vi "LJM_eAddresses2D.vi"(0 "Handle In":i32, 1 "NumFrames (Auto-Detect)":i32=-1, 5 "aAddresses":i32[](array[numeric]), 7 "aTypes":i32[](array[numeric]), 9 "aValuesIn":dbl[][](array[numeric]) format="%.2f", 11 "error in":errorcluster, 12 "aWrites":i32[](array[ring]) items=["Read", "Write"], 13 "aNumValues":i32[](array[numeric])) -> (4 "Handle Out":i32, 10 "aValuesOut":dbl[][](array[numeric]) format="%.2f", 14 "ErrorAddress":i32, 15 "error out":errorcluster)   [LabVIEW 2020]
uses:
  Library/Frameworks/LabJackM.framework
panel:
  # "1/20/2015:  Default value of NumFrames changed to -1 which\nequates to Auto-Detect.  If NumFrames = -1, then the NumFrames\ncontrol is ignored and the size of aNames/aAddresses is used to\ndetermine how many frames there are."
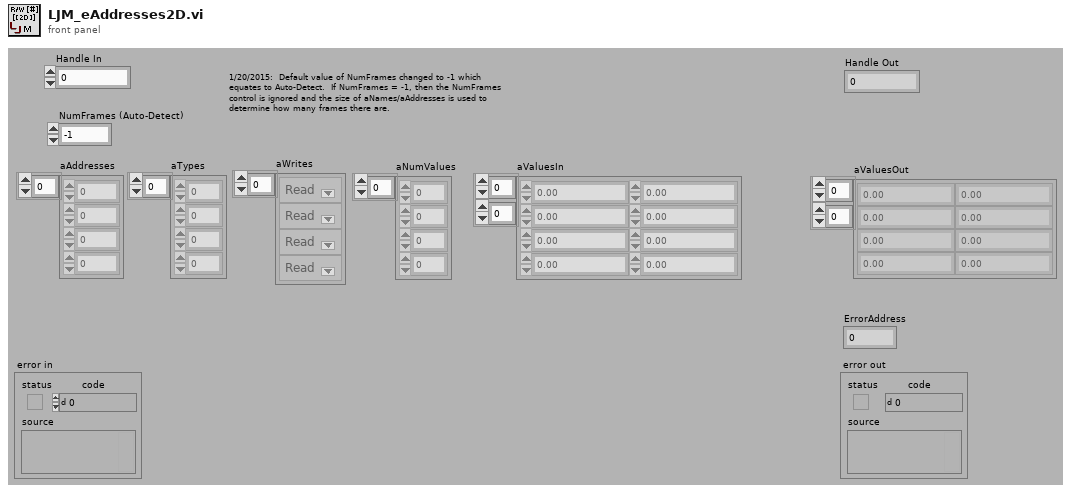
[diagram p1: front panel]
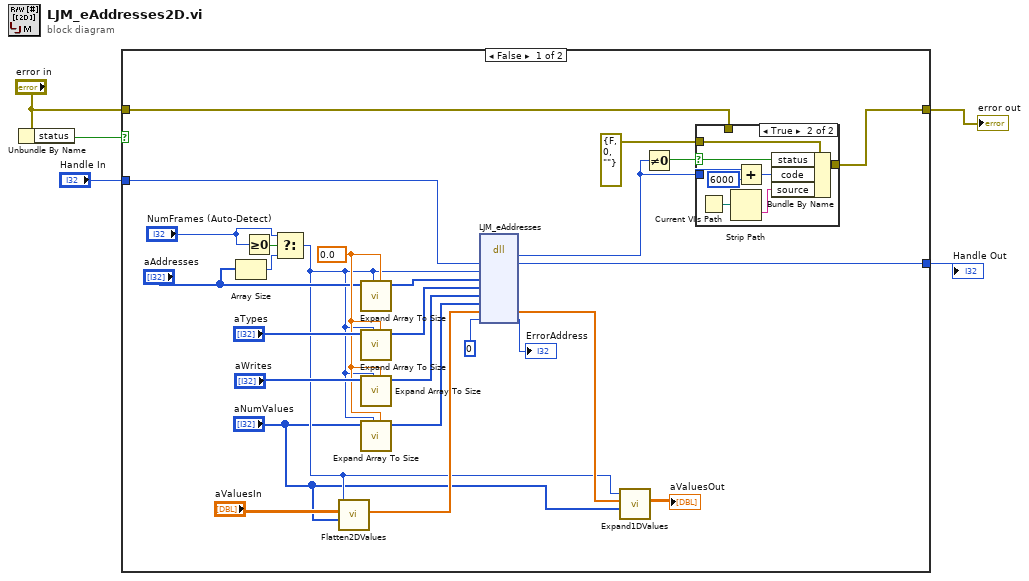
[diagram p0: block diagram]
diagram:
  n1 = Unbundle By Name("error in") -> ("status"=w5:bool)
  n2 = case shown="False" w5 {
    tunnel: "error in" -> [w28 w42]
    tunnel: [w27 w42] -> w3
    tunnel: [w13 w41] -> w2
    tunnel: "Handle In" -> [w12 w41]
    frame False {
      w18 = 0.0 ("Default Value")
      n3 = Array Size(array="aAddresses") -> (size(s)=w11:i32)
      n4 = Greater Or Equal To 0?(x="NumFrames (Auto-Detect)") -> (x >= 0?=w10:bool)
      n5 = Select(t="NumFrames (Auto-Detect)", s=w10, f=w11) -> (s? t:f=w7:i32)
      n6 = call "Flatten2DValues.vi"("NumValues"="aNumValues", "Values 2D"="aValuesIn", "NumFrames"=w7) -> ("Values 1D"=w16:dbl[])  [unwired: 8 in]
      n7 = call "Expand Array To Size.vi"("Default Value"=w18, "# Elements"=w7, "I32 Array In"="aAddresses") -> ("I32 Array Out"=w26:i32[])  [unwired: 4 in, 4 out]
      n8 = call "Expand Array To Size.vi"("Default Value"=w18, "# Elements"=w7, "I32 Array In"="aTypes") -> ("I32 Array Out"=w24:i32[])  [unwired: 4 in, 4 out]
      n9 = call "Expand Array To Size.vi"("Default Value"=w18, "# Elements"=w7, "I32 Array In"="aWrites") -> ("I32 Array Out"=w22:i32[])  [unwired: 4 in, 4 out]
      n10 = call "Expand Array To Size.vi"("Default Value"=w18, "# Elements"=w7, "I32 Array In"="aNumValues") -> ("I32 Array Out"=w21:i32[])  [unwired: 4 in, 4 out]
      n11 = dll-call lib="Library/Frameworks/LabJackM.framework" fn="LJM_eAddresses"("Handle"=w12, "NumFrames"=w7, "aAddresses"=w26, "aTypes"=w24, "aWrites"=w22, "aNumValues"=w21, "aValues"=w16, "ErrorFrame"=u32 0) -> ("return type"=w31:i32, "Handle"=w13:i32, "aValues"=w15:dbl[], "ErrorFrame"=→"ErrorAddress":i32)  [unwired: 8 in, 2 out]
      n12 = call "Expand1DValues.vi"("NumValues"="aNumValues", "Values 1D"=w15, "NumFrames"=w7) -> ("Values 2D"=→"aValuesOut":dbl[][])  [unwired: 8 in]
      n13 = Not Equal To 0?(x=w31) -> (x != 0?=w30:bool)
      n14 = case shown="True" w30 {
        selector: w30 -> [_ w39]
        tunnel: [w32 w40] -> w27
        tunnel: errorcluster {"status"=FALSE, "code"=0, "source"=""} ("error IO") -> [_ w38]
        tunnel: w31 -> [_ w34]
        tunnel: w28 -> [w32 _]
        frame False {
        }
        frame True {
          n15 = Current VI's Path() -> (path=w36:path)
          n16 = Strip Path(path=w36) -> (name=w37:string)  [unwired: 1 out]
          n17 = Add(x=w34, y=6000) -> (x+y=w35:i32)
          n18 = Bundle By Name(cluster=w38, "status"=w39, "code"=w35, "source"=w37) -> (w40:errorcluster)
        }
      }
    }
    frame True {
    }
  }
  "error out" <- w3
  "Handle Out" <- w2
